vi "DrawRectangle.vi"(11 "Zone.lvclass in":refnum<class "Zone.lvclass">) -> (3 "Zone.lvclass out":refnum<class "Zone.lvclass">)   [LabVIEW 2021, in "Zone.lvclass"]
uses:
  LabVIEW Data/Zone/Zone.lvclass
  LabVIEW Data/Zone/Zone.lvclass/Zone.ctl
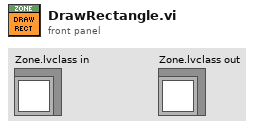
[diagram p1: front panel]
types:
  T1 = cluster{"Width":i16, "Style":enum32{"Solid", "Dash", "Dot", "DashDot", "DashDotDot"}}
  T2 = cluster{"left":i16, "top":i16, "right":i16, "bottom":i16}
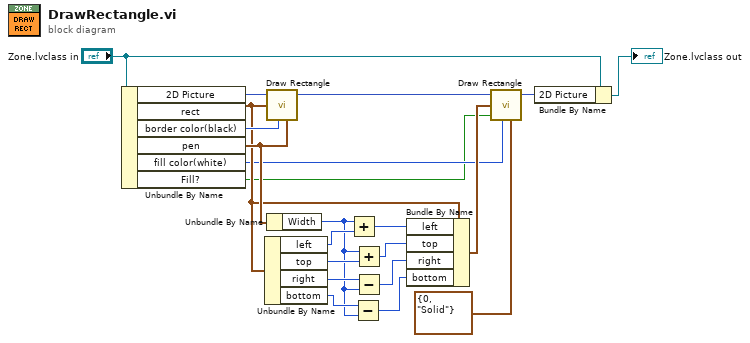
[diagram p0: block diagram]
diagram:
  n1 = Unbundle By Name("Zone.lvclass in") -> ("2D Picture"=w21:picture, "rect"=w6:T2, "border color(black)"=w18:u32, "pen"=w9:T1, "fill color(white)"=w3:u32, "Fill?"=w1:bool)
  n2 = Unbundle By Name(w6) -> ("left"=w10:i16, "top"=w11:i16, "right"=w12:i16, "bottom"=w13:i16)
  n3 = call <vilib>:"Draw Rectangle.vi"("picture"=w21, "rect"=w6, "color(black)"=w18, "pen"=w9) -> ("new picture"=w7:picture)  [unwired: 5 in]
  n4 = Unbundle By Name(w9) -> ("Width"=w8:i16)
  n5 = Add(x=w8, y=w10) -> (x+y=w14:i16)
  n6 = Subtract(x=w13, y=w8) -> (x-y=w17:i16)
  n7 = Add(x=w8, y=w11) -> (x+y=w15:i16)
  n8 = Subtract(x=w12, y=w8) -> (x-y=w16:i16)
  n9 = Bundle By Name(cluster=w6, "left"=w14, "top"=w15, "right"=w16, "bottom"=w17) -> (w5:T2)
  n10 = call <vilib>:"Draw Rectangle.vi"("picture"=w7, "rect"=w5, "fill?(F)"=w1, "color(black)"=w3, "pen"=T1 {"Width"=0, "Style"=enum."Solid"}) -> ("new picture"=w4:picture)  [unwired: 4 in]
  n11 = Bundle By Name(cluster="Zone.lvclass in", "2D Picture"=w4) -> (→"Zone.lvclass out":refnum<class "Zone.lvclass">)
